vi "Actor Core.vi"(8 "error in":errorcluster, 11 "Nested in":refnum<class "Monedas.lvclass">) -> (0 "error out":errorcluster, 3 "Actor out":refnum<class "Actor.lvclass">)   [LabVIEW 2020, in "Monedas.lvlib" / "Monedas.lvclass"]
doc: "(<B>Filename</B>: Actor Framework.lvlib:Actor.lvclass:Actor Core.vi)\n\nReceives messages to the actor, reacts to them, and initiates any error handling that may shut the actor down.\n\nDescendant classes may override this VI to append parallel tasks for the actor to complete while it handles messages. Overrides use the Call Parent Method node."
uses:
  Monedas.lvclass
  <vilib>/ActorFramework/Actor/Actor.lvclass
  <vilib>/ActorFramework/Stop Msg/Stop Msg.lvclass
  C:/Program Files (x86)/National Instruments/LabVIEW 2020/vi.lib/ActorFramework/Actor/Actor.lvclass
  C:/Users/Pablo/AF-Machine-Vending-/AF Machine/Monedas/Monedas.lvclass
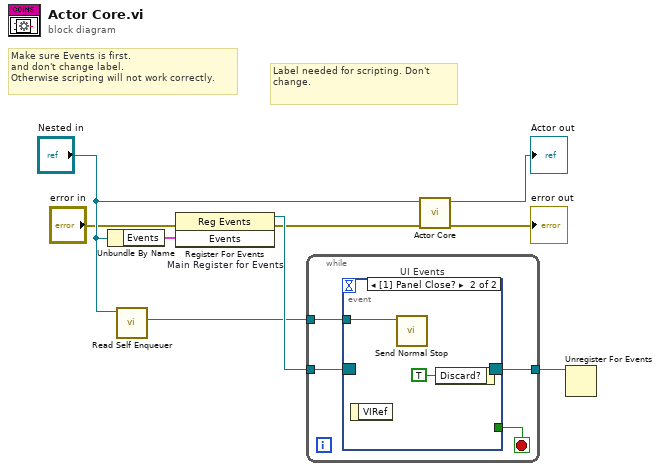
[diagram p0: block diagram]
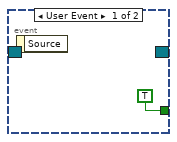
[diagram p2: hidden frame]
diagram:
  # "Label needed for scripting. Don't change."
  # "Make sure Events is first.\nand don't change label.\nOtherwise scripting will not work correctly."
  n1 = Unbundle By Name("Nested in") -> ("Events"=w6:cluster{"Stop":refnum<user-event>})
  n2 = call <vilib>:"Read Self Enqueuer.vi"("Actor"="Nested in") -> ("Self Enqueuer"=w3:refnum<class "Message Enqueuer.lvclass">)  [unwired: 10 in]
  n3 = register-events "Main Register for Events"(error in="error in", w6) -> (reference out=w7:refnum<event-registration>, error out=w1:errorcluster)  [unwired: 1 in]
  n4 = while {
    tunnel: w7 -> [w13]
    tunnel: [w11] -> w5
    tunnel: w3 -> [w10]
    stop <- w12 stop-if-true
    n5 = event "UI Events" shown="[1] Panel Close?" {
      selector: w13 -> [_ _]
      dyn-events: [_ _] -> w11
      timeout: _ -> [_ _]
      tunnel: [TRUE _] -> w12
      tunnel: w10 -> [_ w15]
      event User Event {
        n6 = event-data() -> ()  [unwired: 1 in, 1 out]
      }
      event Panel Close? {
        n7 = event-data() -> ()  [unwired: 1 in, 1 out]
        n8 = call <vilib>:"Send Normal Stop.vi"("Message Enqueuer"=w15) -> ()  [unwired: 10 in, 1 out]
        n9 = event-data("Discard?"=TRUE) -> ()  [unwired: 1 in, 1 out]
      }
    }
  }
  n10 = call-parent "Actor Core.vi"("error in"=w1, "Actor in"="Nested in") -> ("error out"=→"error out":errorcluster, "Actor out"=→"Actor out":refnum<class "Actor.lvclass">)  [unwired: 8 in]
  n11 = Unregister For Events(event registration refnum=w5) -> ()  [unwired: 1 in, 1 out]
